vi "Modtag_Helt_billede.vi"() -> ()   [LabVIEW 2018]
uses:
  <vilib>/myRIO/Instrument Drivers/Onboard IO/UART/typedef/VISA Configuration.ctl
  <vilib>/Instr/_visa.llb/VISA Configure Serial Port (Instr).vi
  <vilib>/myRIO/Express VI/Onboard IO/UART/UART Express VI.xnode
  <vilib>/myRIO/Instrument Drivers/Onboard IO/UART/UART.lvlib
panel:
  out "Characters Read":string
  out "Intensity Graph 7":u8[][](graph)
  in  "stop":bool
  out "array":u8[][](array[numeric])
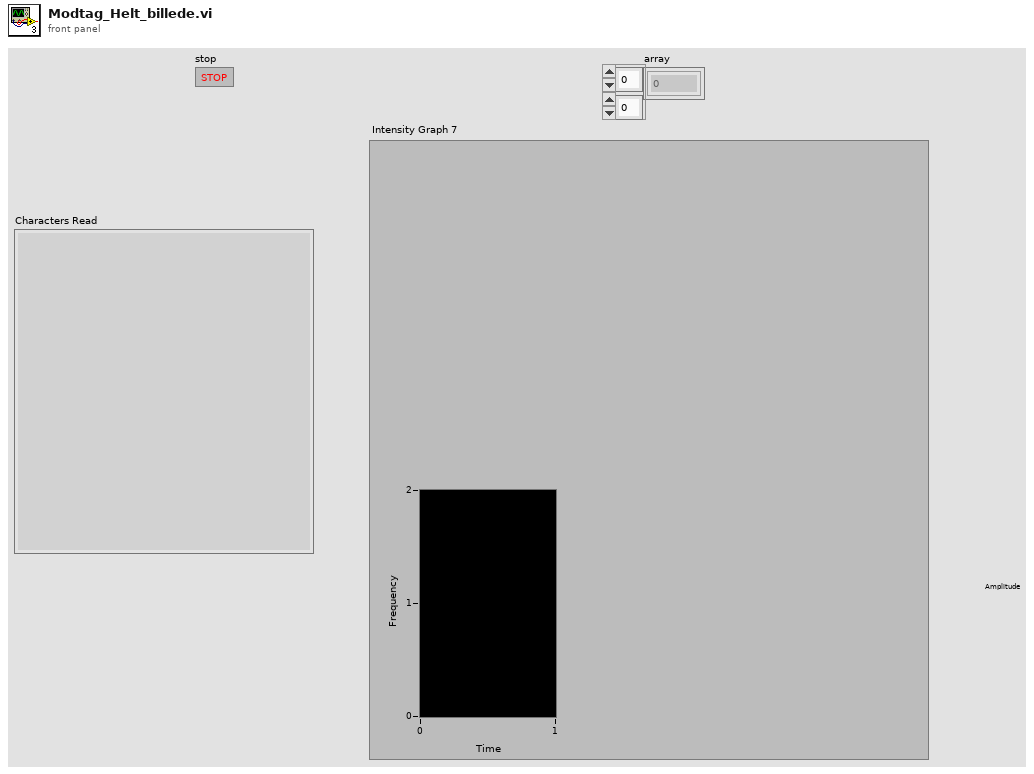
[diagram p1: front panel]
types:
  T1 = typedef "UART.lvlib/VISA Configuration.ctl" = cluster{"baud rate (9600)":u32, "data bits (8)":u16, "parity (0:none)":enum16{"None", "Odd", "Even", "Mark", "Space"}, "stop bits (10: 1 bit)":u16, "flow control (0:none)":u16, "termination char\n(0xA = '\\n' = LF) ":u8, "Enable Termination\nChar (T)":bool, "timeout (10sec)":u32}
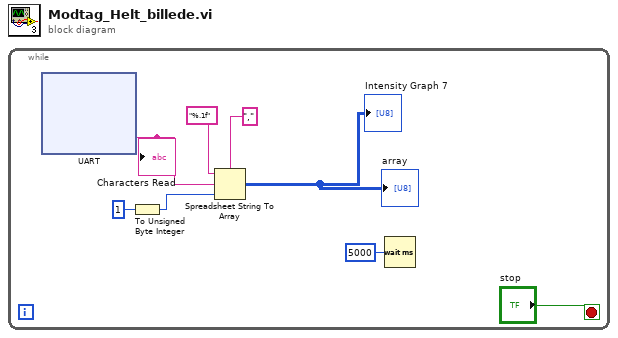
[diagram p0: block diagram]
diagram:
  n1 = while {
    stop <- "stop" stop-if-true
    n2 = xnode "UART"() -> ("Characters Read"=w8:string)  [unwired: 1 in, 1 out]
    "Characters Read" <- w8
    n3 = To Unsigned Byte Integer(number=u8 1) -> (unsigned 8bit integer=w4:u8)
    n4 = Spreadsheet String To Array(delimiter (Tab)=",", format string="%.1f", spreadsheet string=w8, array type (2D Dbl)=w4) -> (array=→"array" →"Intensity Graph 7":u8[][])
    n5 = Wait (ms)(milliseconds to wait=u32 5000) -> ()  [unwired: 1 out]
  }
